vi "DWE Search 2D Array (I32).vi"(10 "Element":i32, 11 "Array":i32[][](array[numeric])) -> (3 "Locations":i32[][](array[numeric]))   [LabVIEW 2023]
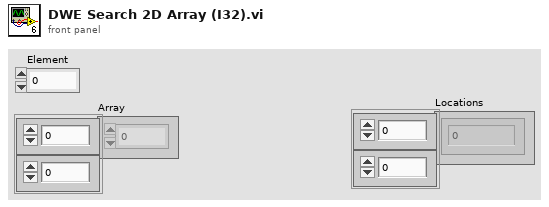
[diagram p1: front panel]
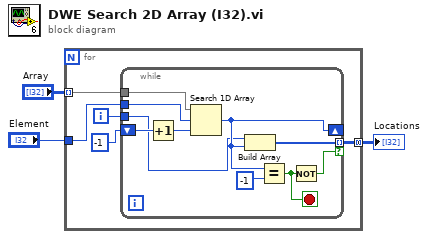
[diagram p0: block diagram]
diagram:
  n1 = for {
    tunnel: "Array" -> [w8] mode=indexing
    tunnel: "Element" -> [w7]
    tunnel: [w5] -> w1 mode=concatenating
    i -> [w6]
    n2 = while {
      tunnel: w8 -> [w18]
      tunnel: w7 -> [w17]
      shift-right: [w14] -> _
      shift-left: -1 ("index of element") -> [w16]
      tunnel: w6 -> [w13]
      tunnel: [w12] -> w5 mode=indexing if=w9
      stop <- w10 stop-if-true
      n3 = Increment(x=w16) -> (x+1=w11:i32)
      n4 = Search 1D Array(1D array=w18, element=w17, start index (0)=w11) -> (index of element=w14:i32)
      n5 = Build Array(w13, w14) -> (w12:i32[])
      n6 = Equal?(x=w14, y=-1) -> (x = y?=w10:bool)
      n7 = Not(x=w10) -> (.not. x?=w9:bool)
    }
  }
  "Locations" <- w1
